vi "Trace Message.vi"(8 "error in (no error)":errorcluster, 10 "Message":string, 11 "System in":refnum<class "System.lvclass">) -> (0 "error out":errorcluster, 3 "System out":refnum<class "System.lvclass">)   [LabVIEW 2013, in "System.lvclass"]
uses:
  System.lvclass
  System.lvclass/System.ctl
  TraceMessage/Trace.lvclass
  Tracer Messages/Record TraceMessage Msg/Log Trace Msg.lvclass
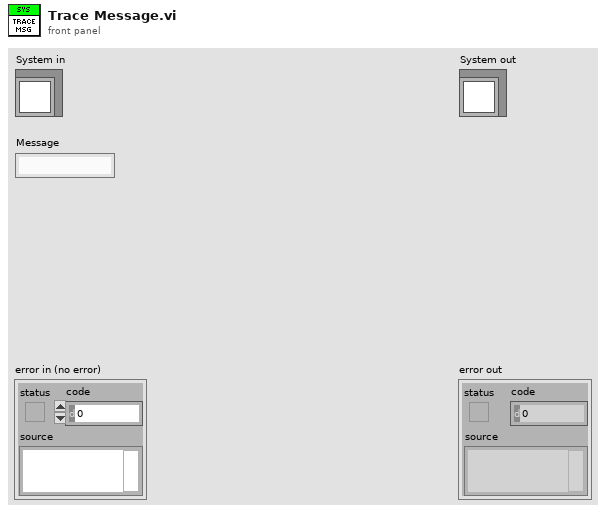
[diagram p1: front panel]
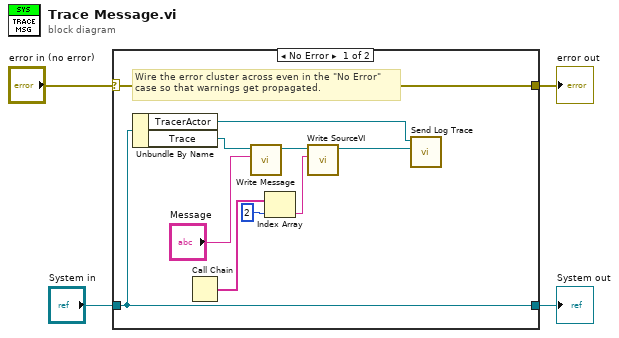
[diagram p0: block diagram]
diagram:
  n1 = case shown="No Error" "error in (no error)" {
    selector: "error in (no error)" -> [w14 w16]
    tunnel: [w14 w16] -> w3
    tunnel: [w12 w15] -> w1
    tunnel: "System in" -> [w12 w15]
    frame No Error {
      # "Wire the error cluster across even in the \"No Error\"\ncase so that warnings get propagated."
      n2 = Unbundle By Name(w12) -> ("TracerActor"=w11:refnum<class "Message Enqueuer.lvclass">, "Trace"=w6:refnum<class "Trace.lvclass">)
      n3 = Call Chain() -> (call chain=w9:string[])
      n4 = call-dynamic "Write Message.vi"("Message"="Message", "TraceMessage in"=w6) -> ("TraceMessage out"=w7:refnum<class "Trace.lvclass">)  [unwired: 8 in, 1 out]
      n5 = Index Array(array=w9, index=2) -> (element=w8:string)
      n6 = call-dynamic "Write SourceVI.vi"("SourceVI"=w8, "Trace in"=w7) -> ("Trace out"=w10:refnum<class "Trace.lvclass">)  [unwired: 8 in, 1 out]
      n7 = call "Send Log Trace.vi"("Trace"=w10, "Message Enqueuer"=w11) -> ()  [unwired: 8 in, 2 out]
    }
    frame Error {
    }
  }
  "error out" <- w3
  "System out" <- w1
